vi "exercicios13_queue.vi"() -> ()   [LabVIEW 2018]
panel:
  out "Numeric":i32
  out "LED 3":bool
  out "LED 2":bool
  out "LED 1":bool
  out "Histórico:":string
  in  "?":bool
  in  "Comandos:":string
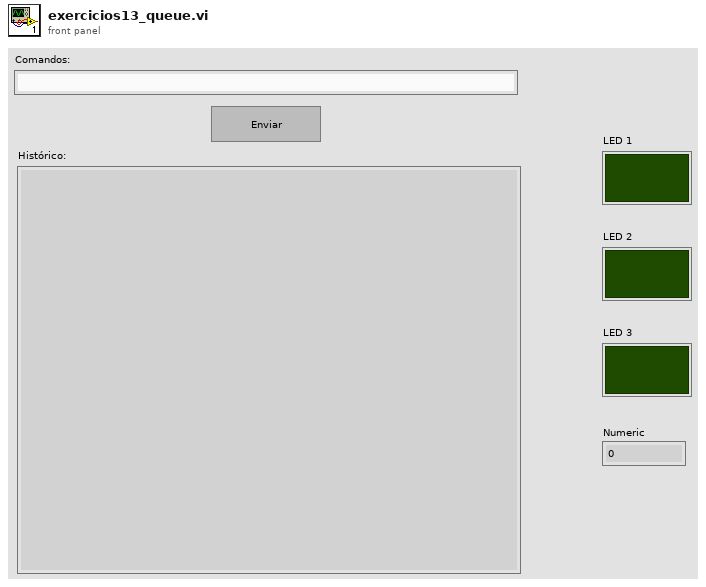
[diagram p1: front panel]
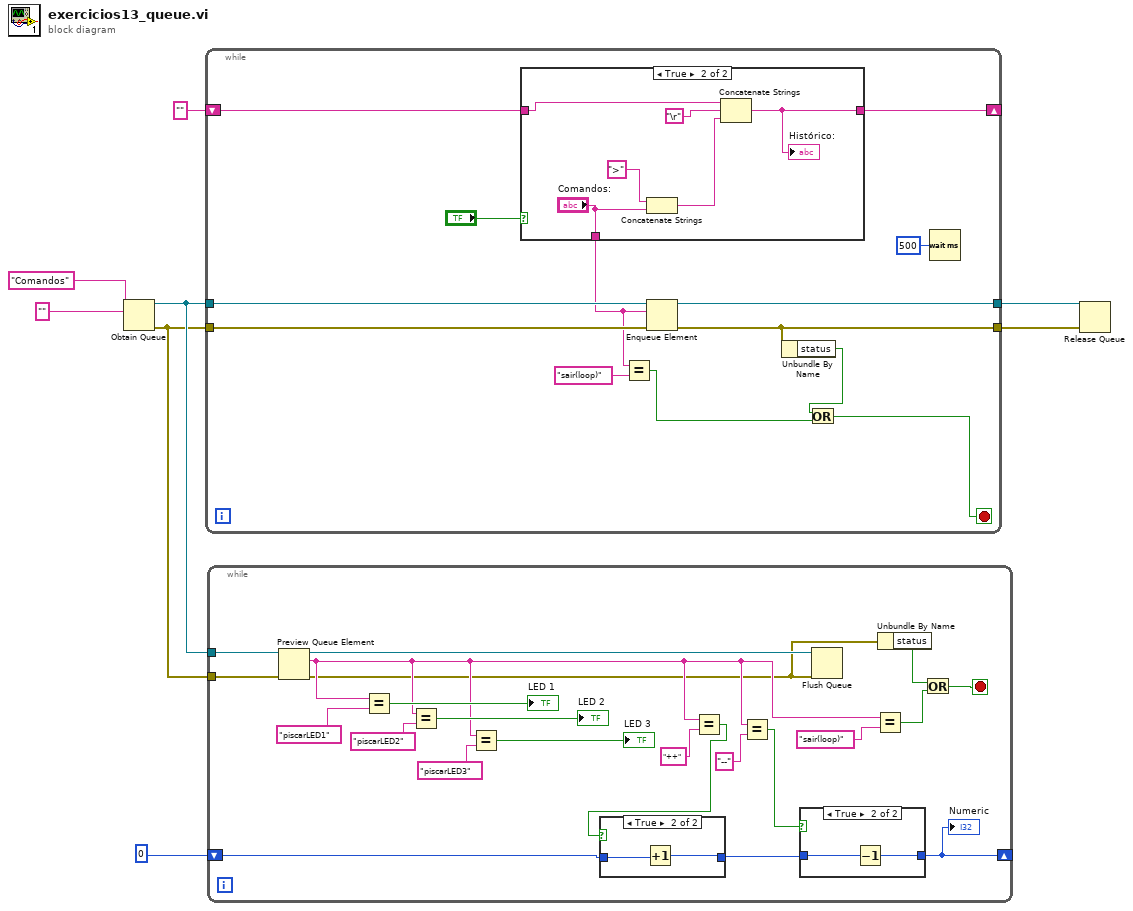
[diagram p0: block diagram]
diagram:
  n1 = Obtain Queue(name (unnamed)="Comandos", element data type="") -> (queue out=w3:refnum<queue>, error out=w2:errorcluster)  [unwired: 3 in, 1 out]
  n2 = while {
    tunnel: w3 -> [w21]
    tunnel: w2 -> [w20]
    shift-right: [w16] -> _
    shift-left: "" -> [w17]
    tunnel: [w18] -> w5
    tunnel: [w13] -> w4
    stop <- w10 stop-if-true
    n3 = case shown="True" "?" {
      tunnel: [_ "Comandos:"] -> w15
      tunnel: [w22 w23] -> w16
      tunnel: w17 -> [w22 w26]
      frame False {
      }
      frame True {
        n4 = Concatenate Strings(">" ("string"), "Comandos:") -> (w24:string)
        n5 = Concatenate Strings(w26, "\r", w24) -> (w23:string)
        "Histórico:" <- w23
      }
    }
    n6 = Equal?(x=w15, y="sair(loop)") -> (x = y?=w11:bool)
    n7 = Enqueue Element(queue=w21, element=w15, error in (no error)=w20) -> (queue out=w18:refnum<queue>, error out=w13:errorcluster)  [unwired: 1 in, 1 out]
    n8 = Unbundle By Name(w13) -> ("status"=w12:bool)
    n9 = Or(x=w12, y=w11) -> (x .or. y?=w10:bool)
    n10 = Wait (ms)(milliseconds to wait=u32 500) -> ()  [unwired: 1 out]
  }
  n11 = while {
    tunnel: w3 -> [w50]
    tunnel: w2 -> [w49]
    shift-right: [w29] -> _
    shift-left: 0 -> [w36]
    stop <- w30 stop-if-true
    n12 = Preview Queue Element(queue=w50, error in (no error)=w49) -> (queue out=w48:refnum<queue>, element=w35:string, error out=w33:errorcluster)  [unwired: 1 in, 1 out]
    n13 = Equal?(x=w35, y="piscarLED1") -> (x = y?=→"LED 1":bool)
    n14 = Equal?(x=w35, y="piscarLED2") -> (x = y?=→"LED 2":bool)
    n15 = Equal?(x=w35, y="piscarLED3") -> (x = y?=→"LED 3":bool)
    n16 = Equal?(x=w35, y="++") -> (x = y?=w39:bool)
    n17 = case shown="True" w39 {
      tunnel: [w54 w55] -> w37
      tunnel: w36 -> [w54 w56]
      frame False {
      }
      frame True {
        n18 = Increment(x=w56) -> (x+1=w55:i32)
      }
    }
    n19 = Equal?(x=w35, y="--") -> (x = y?=w38:bool)
    n20 = case shown="True" w38 {
      tunnel: w37 -> [w51 w53]
      tunnel: [w51 w52] -> w29
      frame False {
      }
      frame True {
        n21 = Decrement(x=w53) -> (x-1=w52:i32)
      }
    }
    "Numeric" <- w29
    n22 = Flush Queue(queue=w48, error in (no error)=w33) -> ()  [unwired: 3 out]
    n23 = Equal?(x=w35, y="sair(loop)") -> (x = y?=w31:bool)
    n24 = Unbundle By Name(w33) -> ("status"=w32:bool)
    n25 = Or(x=w32, y=w31) -> (x .or. y?=w30:bool)
  }
  n26 = Release Queue(queue=w5, error in (no error)=w4) -> ()  [unwired: 1 in, 3 out]
